vi "Main.vi"() -> ()   [LabVIEW 2017]
uses:
  <userlib>/_NEVSTOP/Communicable State Machine(CSM)/_Polymophic/Add State(s) to Queue By BOOL(Element).vi
  9fd6aee3-8c61-4172-ac23-ecfb0dc55d82.vi
  757b7255-c684-43ce-af59-1acc32dadd6e.vi
  <vilib>/Analysis/2dsp.llb/Real FFT.vi
  <userlib>/_NEVSTOP/Communicable State Machine(CSM)/_Support/CSMQ/_Obtain CSMQ.vi
  <userlib>/_NEVSTOP/Communicable State Machine(CSM)/_Support/FGV-BroadcastRegistry/Cache-Broadcast Registry Search Result.vi
  <userlib>/_NEVSTOP/Communicable State Machine(CSM)/AdvanceAPI/CSM - Unregister Status Change.vi
  <userlib>/_NEVSTOP/Communicable State Machine(CSM)/_Support/CSMQ/_Create Resp Queue.vi
  <userlib>/_NEVSTOP/Communicable State Machine(CSM)/_Support/CSMQ/_Unlock CSMQ.vi
  <userlib>/_NEVSTOP/Communicable State Machine(CSM)/_Support/CSMQ/_Lock State CSMQ.vi
  <userlib>/_NEVSTOP/Communicable State Machine(CSM)/_Support/CSMQ/_Release CSMQ.vi
  <userlib>/_NEVSTOP/Communicable State Machine(CSM)/AdvanceAPI/CSM - Make String Arguments Safe.vi
  <userlib>/_NEVSTOP/Communicable State Machine(CSM)/_Support/CSMQ/_Input Name to CSM Mode.vi
  <userlib>/_NEVSTOP/Communicable State Machine(CSM)/Utility/uuid.vi
  <userlib>/_NEVSTOP/Communicable State Machine(CSM)/_Support/KeyWords.vi
  <userlib>/_NEVSTOP/Communicable State Machine(CSM)/_Support/FGV-BroadcastRegistry/FGV-BroadcastRegistry.vi
  MassData-Parameter/_support/FGV-MassData.vi
  <userlib>/_NEVSTOP/Communicable State Machine(CSM)/_Support/GlobalEvent/FGV-GlobalEventRef.vi
  <userlib>/_NEVSTOP/Communicable State Machine(CSM)/_Support/CSMQ/_CSMQFGV.vi
  <userlib>/_NEVSTOP/Communicable State Machine(CSM)/_Support/CSMQ/_Dequeue CSMQ.vi
  <userlib>/_NEVSTOP/Communicable State Machine(CSM)/_Support/CSMQ/_Enqueue CSMQ.vi
  <userlib>/_NEVSTOP/Communicable State Machine(CSM)/_Support/GlobalEvent/FGV-StatusChangeEventRef.vi
  <userlib>/_NEVSTOP/Communicable State Machine(CSM)/_Support/FGV-BroadcastRegistry/global-Broadcast Cache Change Flag.vi
  MassData-Parameter/JKISM++ MassData Parameter Support.lvlib
  <vilib>/Analysis/NI_AALPro.lvlib
  <userlib>/_NEVSTOP/Communicable State Machine(CSM)/Communicable State Machine.lvlib
panel:
  out "fft":dbl[](graph)
  out "read":cluster{dbl, dbl}(slide)={0.0, 6224.489795918367} scale=0.0..1000000.0 scale format="%#_6p"
  out "Write":cluster{dbl, dbl}(slide)={0.0, 6224.489795918367} scale=0.0..1000000.0 scale format="%#_6p"
  in  "Gen?":bool
  in  "DataSize":i32=1000
  out "Waveform Chart":dbl[](graph)
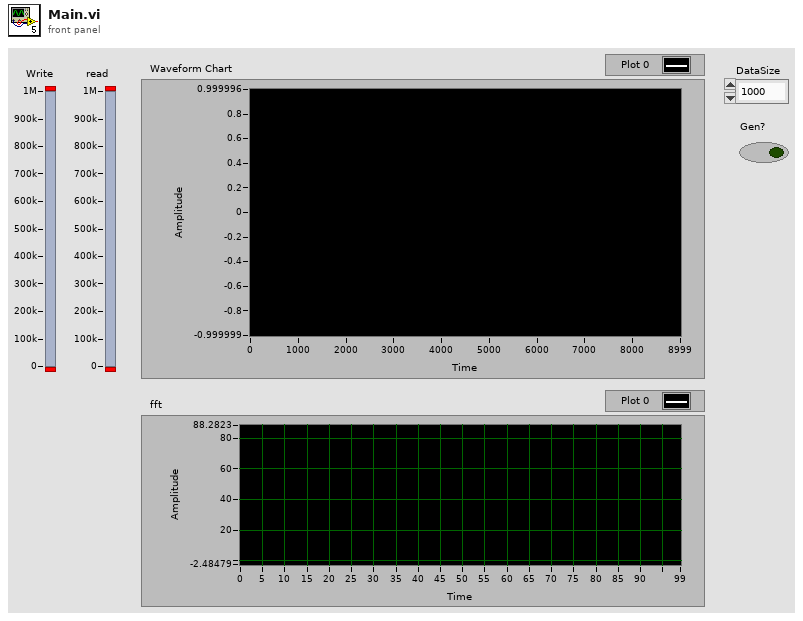
[diagram p1: front panel]
types:
  T1 = enum32{"Invalid", "Standard", "Closed", "Hidden", "Minimized", "Maximized"}
  T2 = enum32{"invalid app kind", "Development System", "Run Time System", "Student Edition", "Embedded LabVIEW", "Evaluation", "Custom"}
  T3 = cluster{"Core":cluster{"Current VI Reference":refnum<vi>, "Close Panel on Exit?":bool}, "Your Boolean data":bool, "Your string data":string}
  T4 = cluster{"Current VI Reference":refnum<vi>, "Close Panel on Exit?":bool}
  T5 = typedef "JKISM++ MassData Parameter Support.lvlib/Def-MassDataOper-Status.ctl" = cluster{"Start":i32, "Size":i32, "Total":i32}
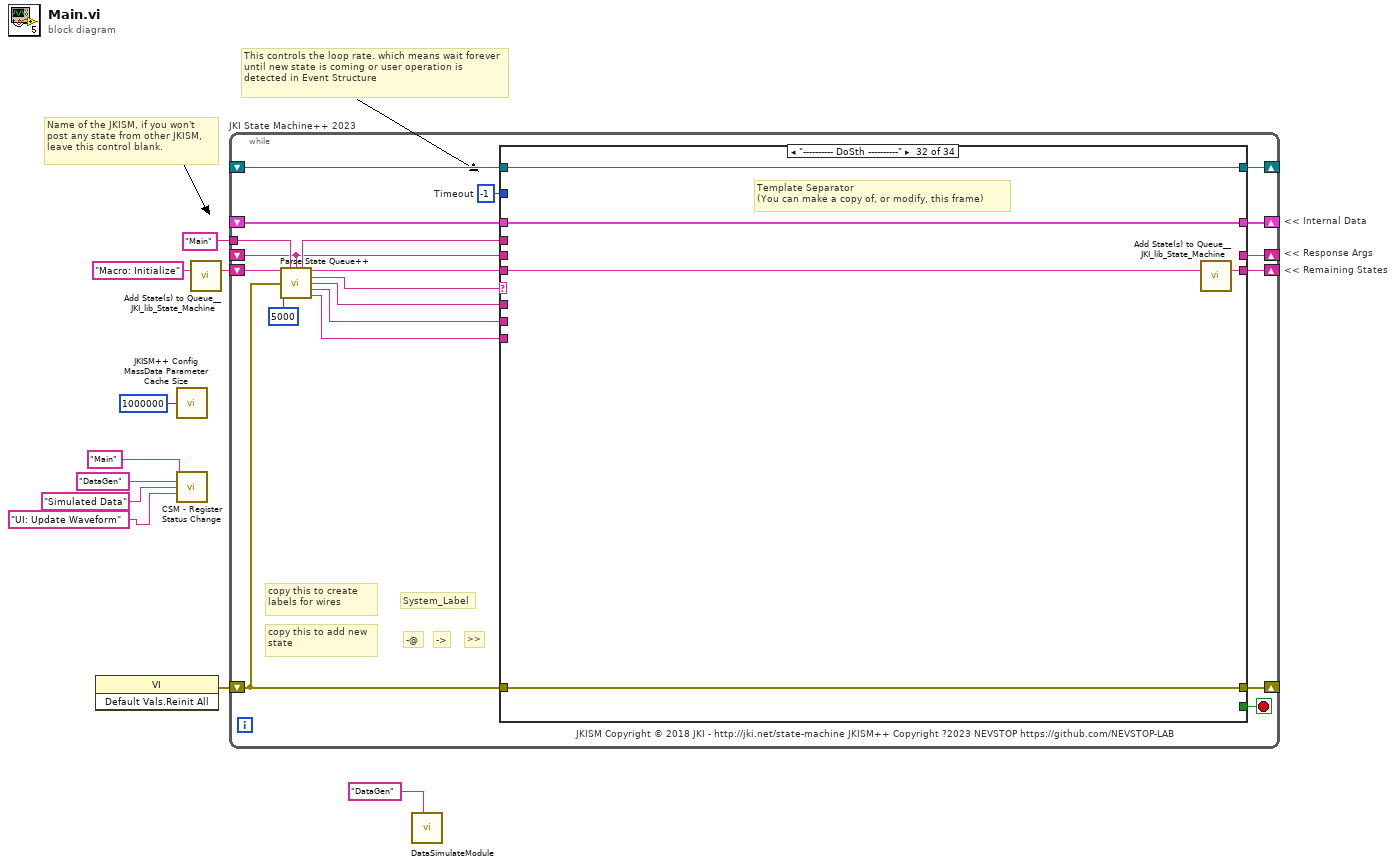
[diagram p0: block diagram]
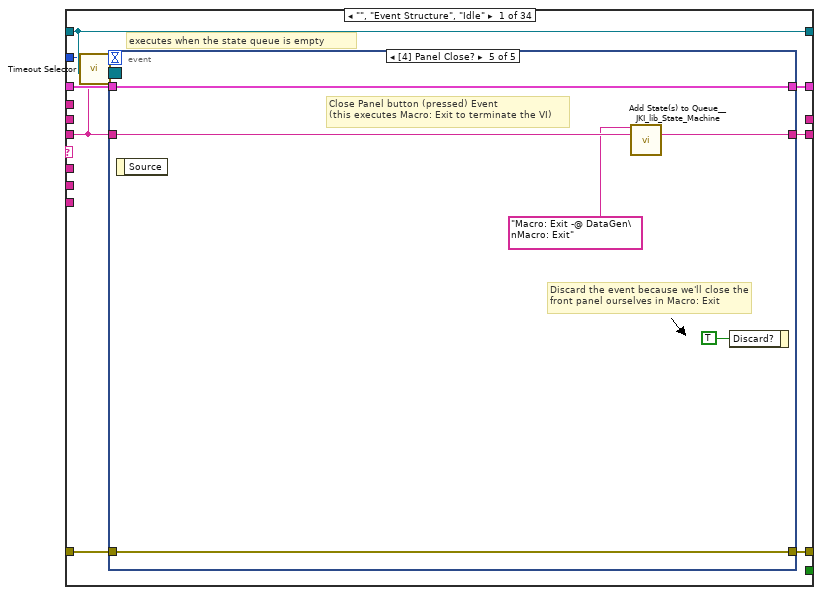
[diagram p2: hidden frame]
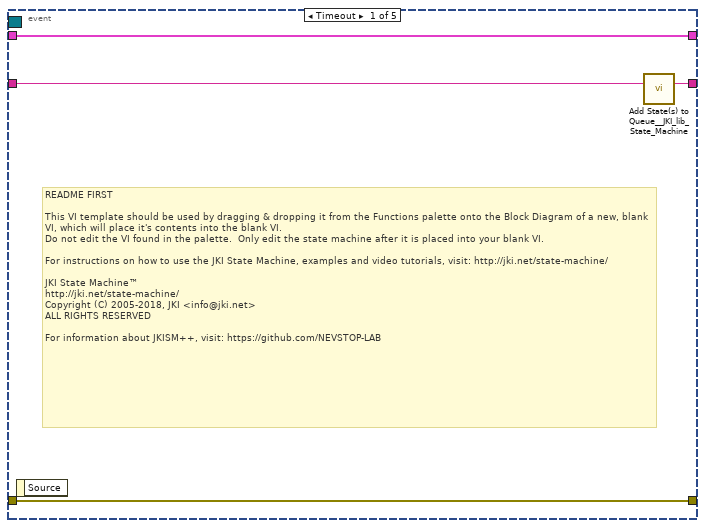
[diagram p3: hidden frame]
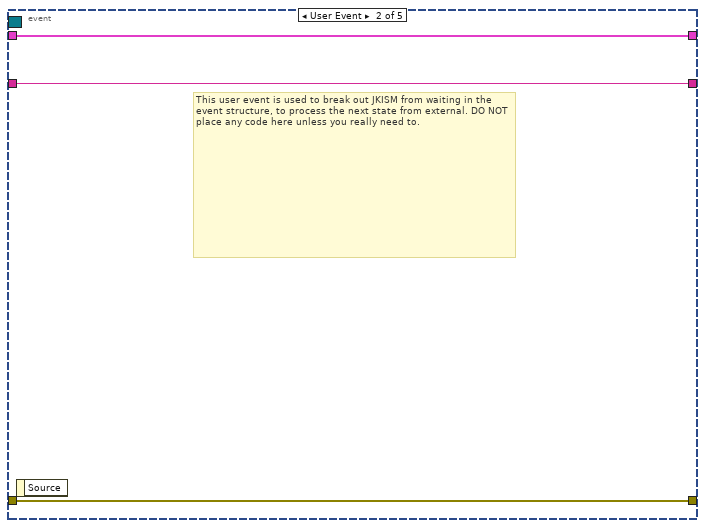
[diagram p4: hidden frame]
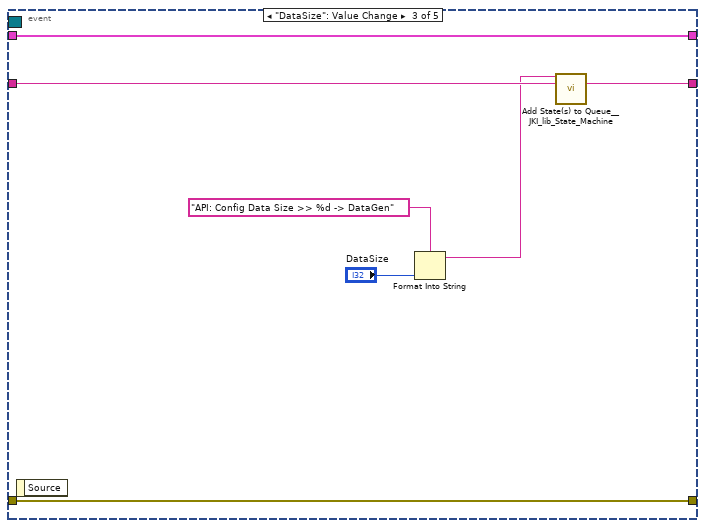
[diagram p5: hidden frame]
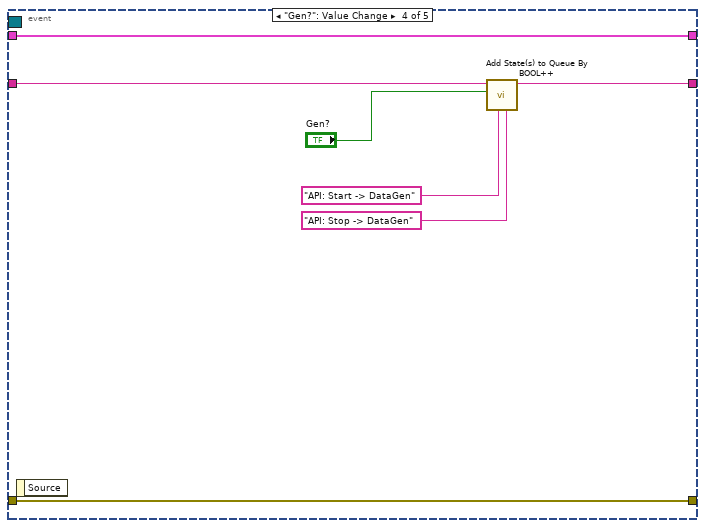
[diagram p6: hidden frame]
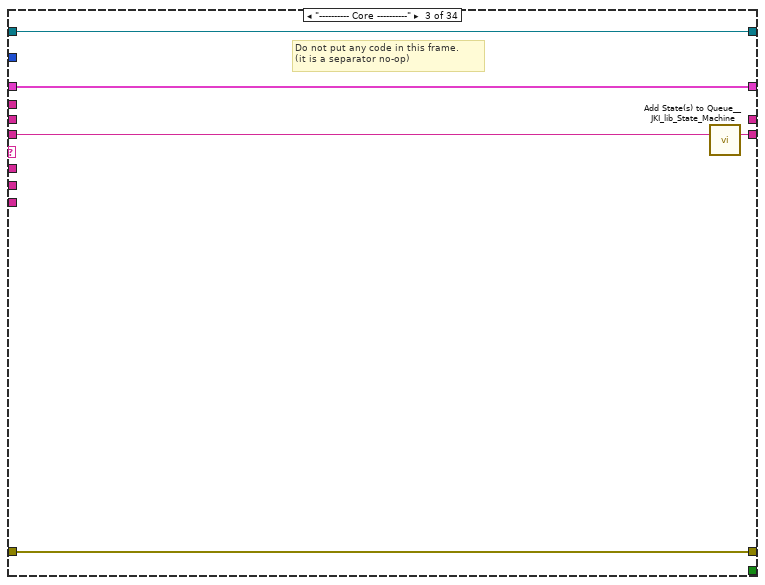
[diagram p8: hidden frame]
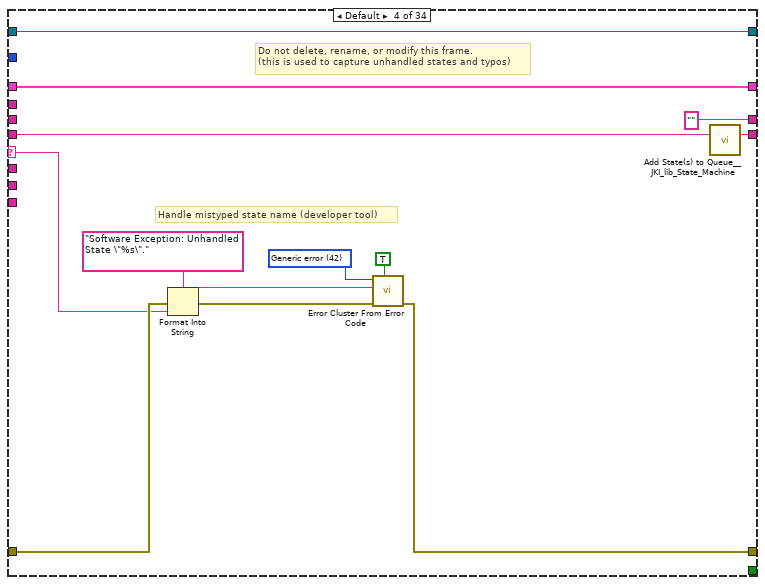
[diagram p9: hidden frame]
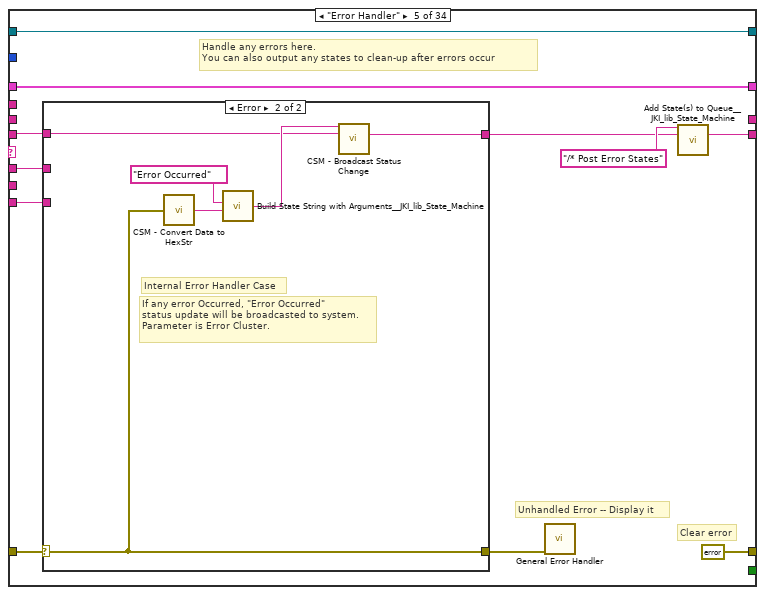
[diagram p10: hidden frame]
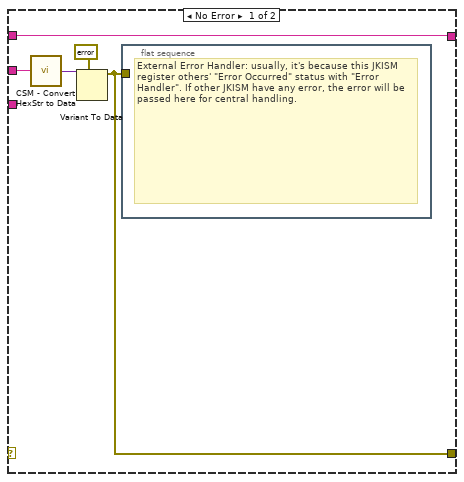
[diagram p11: hidden frame]
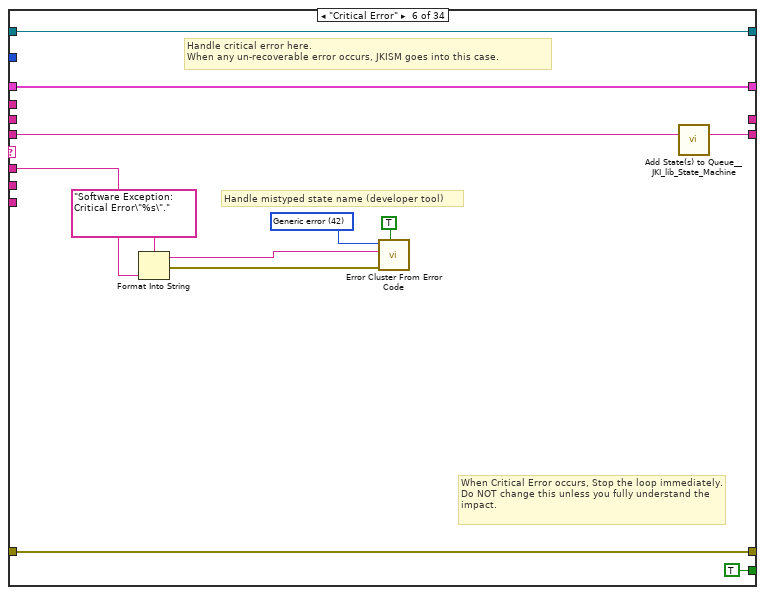
[diagram p12: hidden frame]
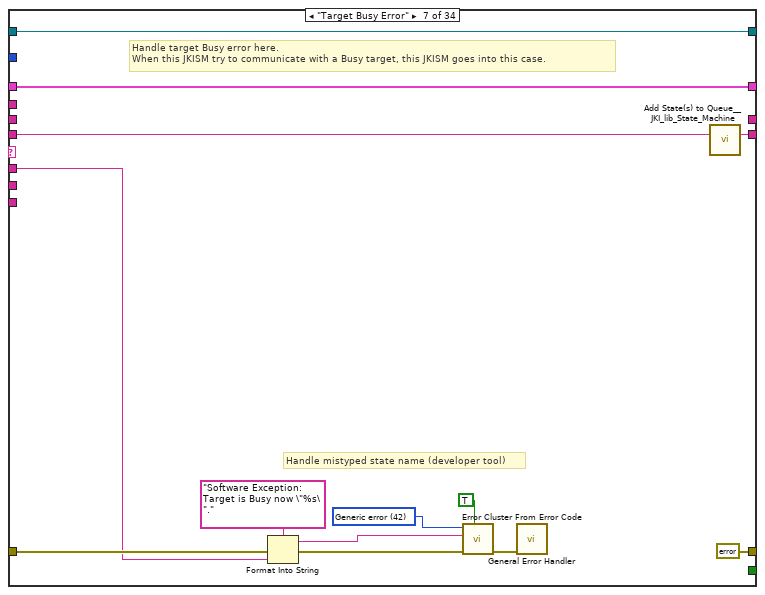
[diagram p13: hidden frame]
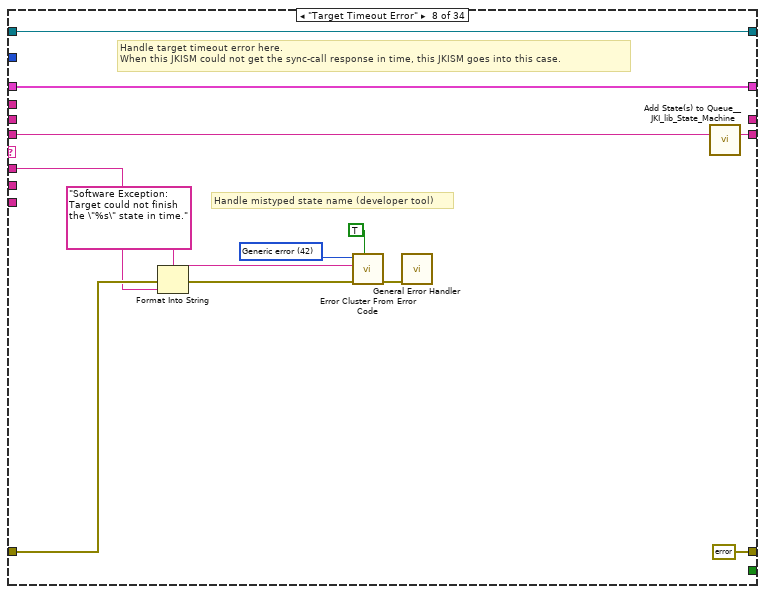
[diagram p14: hidden frame]
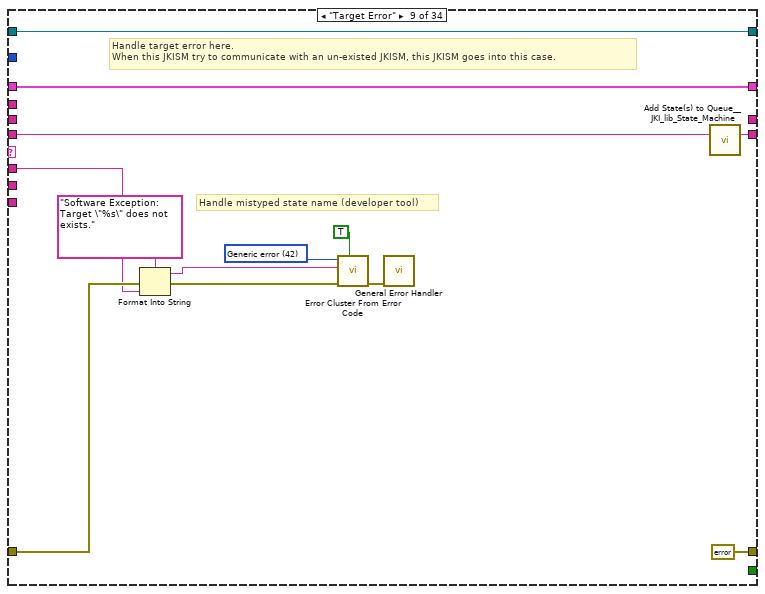
[diagram p15: hidden frame]
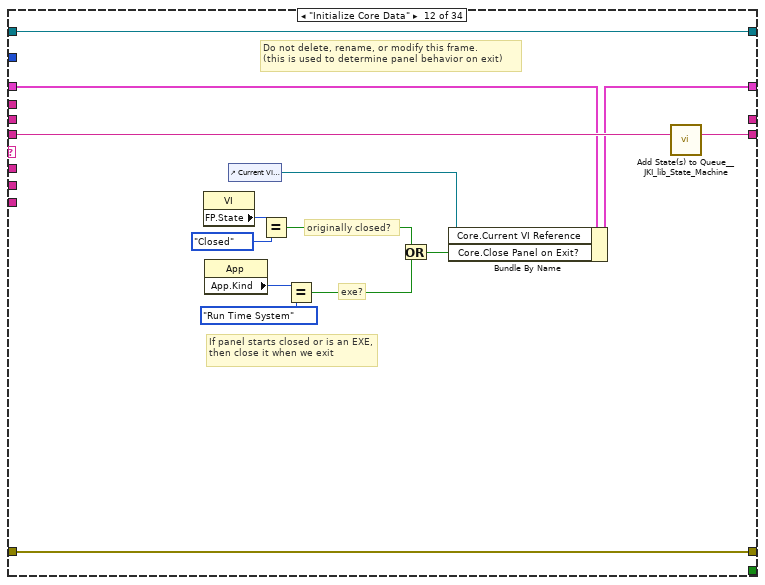
[diagram p18: hidden frame]
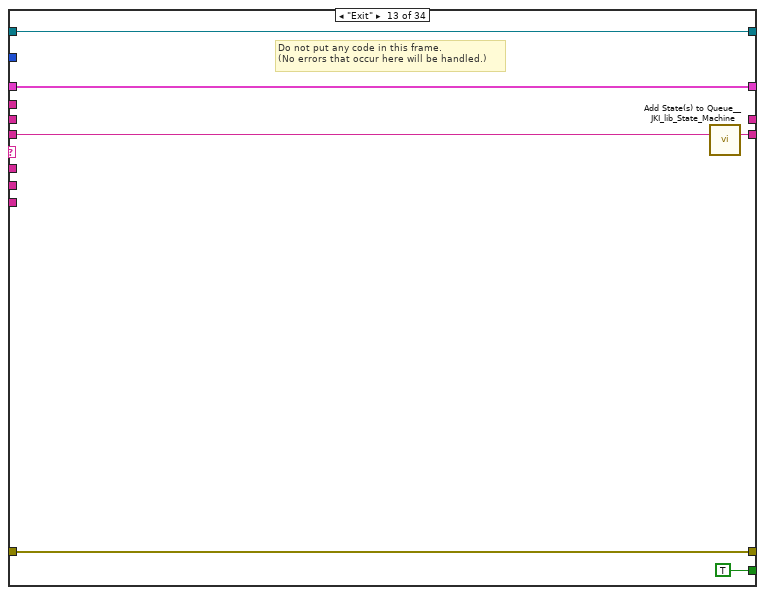
[diagram p19: hidden frame]
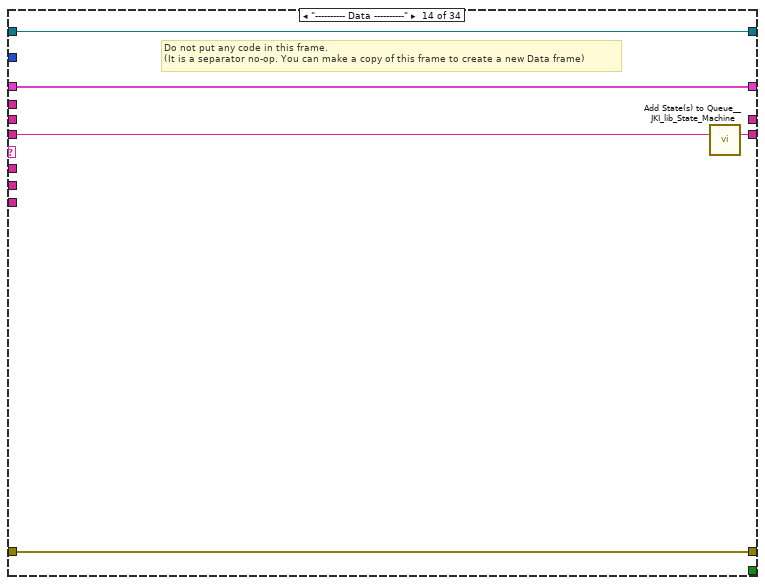
[diagram p20: hidden frame]
diagram:
  # "<< Internal Data"
  # "<< Response Args"
  # "<< Remaining States"
  # "Name of the JKISM, if you won't post any state from other JKISM,  leave this control blank."
  # "This controls the loop rate. which means wait forever until new state is coming or user operation is detected in Event Structure"
  n1 = invoke class="VI" method="Default Vals.Reinit All"() -> (error out=w2:errorcluster)  [unwired: 3 in, 2 out]
  n2 = call "JKISM++ Config MassData Parameter Cache Size.vi"("size(1M)"=1000000) -> ()  [unwired: 9 in]
  n3 = call <userlib>:"CSM - Register Status Change.vi"("CSM Name"="Main" ("JKISM Name"), "Source CSM Name (* as Default)"="DataGen" ("JKISM Name"), "Status"="Simulated Data" ("JKISM Name"), "Response Message (if \"\", same as Source Message)"="UI: Update Waveform" ("JKISM Name")) -> ()  [unwired: 10 in, 2 out]
  n4 = call <vilib>:"Add State(s) to Queue__JKI_lib_State_Machine.vi"("State(s) in (\"\")"="Macro: Initialize") -> ("States Out"=w8:string)  [unwired: 14 in]
  n5 = while "JKI State Machine++ 2023" {
    shift-right: [w25] -> _
    shift-left: _ -> [w24]
    shift-right: [w28] -> _
    shift-left: w2 -> [w22]
    shift-right: [w27] -> _
    shift-left: w8 -> [w29]
    tunnel: "Main" ("Name(\"\" to use uuid)") -> [w17]
    shift-right: [w20] -> _
    shift-left: _ -> [w12]
    shift-right: [w19] -> _
    shift-left: _ -> [w18]
    stop <- w26 stop-if-true
    w23 = -1  # Timeout
    # "JKISM Copyright © 2018 JKI - http://jki.net/state-machine JKISM++ Copyright ?2023 NEVSTOP https://github.com/NEVSTOP-LAB"
    # "copy this to add new state"
    # ">>"
    # "->"
    # "-@"
    # "copy this to create labels for wires"
    # "System_Label"
    n6 = call <userlib>:"Parse State Queue++.vi"("State Queue"=w29, "Name(\"\" to use uuid)"=w17, "Response Arguments"=w12, "Error In (no error)"=w22, "Response Timeout(5000ms)"=5000 ("Response Timeout(1000ms)")) -> ("Name Used"=w13:string, "Remaining States"=w30:string, "Current State"=w16:string, "Arguments"=w11:string, "Argument - State"=w15:string, "From Who"=w14:string)  [unwired: 5 in]
    n7 = case shown="\"---------- DoSth ----------\"" w16 {
      selector: w16 -> [_ _ _ w78 _ _ _ _ _ _ _ _ _ _ _ _ _ _ _ _ _ _ _ _ _ _ _ _ _ _ _ _ _ _]
      tunnel: w30 -> [w31 w69 w75 w82 w92 w120 w125 w143 w156 w164 w168 w183 w189 w194 w202 w209 w214 w220 w224 w230 w240 w247 w263 w334 w352 w361 w367 w373 w384 w387 w392 w398 w404 w410]
      tunnel: w11 -> [_ _ _ _ w90 w113 w127 w139 w152 _ _ _ _ _ _ _ _ _ _ _ _ w242 w257 w329 _ w358 _ _ _ _ _ _ _ _]
      tunnel: w24 -> [w38 w68 w72 w80 w98 w121 w129 w141 w154 w163 w167 w176 w187 w191 _ w204 w211 w219 w223 w227 w238 w245 w259 w338 w351 w360 w364 w370 w381 w386 w391 w395 w401 w407]
      tunnel: [w37 w70 w73 w84 errorcluster {"status"=FALSE, "code"=0, "source"=""} ("error out") w122 errorcluster {"status"=FALSE, "code"=0, "source"=""} ("error out") errorcluster {"status"=FALSE, "code"=0, "source"=""} ("error out") errorcluster {"status"=FALSE, "code"=0, "source"=""} ("error out") w165 w169 w180 w186 w192 w199 w205 w212 w215 w222 w228 w237 w243 w260 w339 w353 w362 w365 w371 w382 w388 w393 w396 w402 w408] -> w28
      tunnel: w22 -> [w36 w70 w73 w83 w96 w122 w131 w144 w157 w165 w169 w180 w186 w192 w199 w206 w212 _ w225 w228 w237 w244 w261 w339 w353 w362 w365 w371 w382 w388 w393 w396 w402 w408]
      tunnel: [w39 w69 w74 w81 w94 w119 w130 w142 w155 w164 w168 w182 w188 w193 w201 w208 w213 w220 w224 w229 w239 w246 w262 w335 w352 w361 w366 w372 w383 w387 w392 w397 w403 w409] -> w27
      tunnel: [_ _ _ _ _ TRUE _ _ _ _ _ _ TRUE _ _ _ _ _ _ _ _ _ _ _ _ _ _ _ _ _ _ _ _ _] -> w26
      tunnel: [w35 w68 w72 w80 w98 w121 w129 w141 w154 w163 w167 w181 w187 w191 w200 w204 w211 w219 w223 w227 w238 w245 w259 w338 w351 w360 w364 w370 w381 w386 w391 w395 w401 w407] -> w25
      tunnel: w23 -> [w33 _ _ _ _ _ _ _ _ _ _ _ _ _ _ _ _ _ _ _ _ _ _ _ _ _ _ _ _ _ _ _ _ _]
      tunnel: w14 -> [_ _ _ _ w89 _ _ _ _ _ _ _ _ _ _ _ _ _ _ _ _ _ _ _ _ _ _ _ _ _ _ _ _ _]
      tunnel: w15 -> [_ _ _ _ _ _ _ _ _ _ _ _ _ _ _ _ _ _ _ _ _ _ _ _ _ _ _ _ _ _ _ _ _ _]
      tunnel: [_ _ _ "" _ _ _ _ _ _ _ _ _ _ _ _ _ _ _ _ _ _ _ _ _ _ _ _ _ _ "API1 Response" _ "DoA Finished" "DoB Finished"] -> w20
      tunnel: [w34 w67 w71 w76 w97 w111 w126 w138 w151 w162 w166 w170 w184 w190 w195 w203 w210 w218 w221 w226 w236 w241 w256 w337 w350 w359 w363 w368 w374 w385 w390 w394 w400 w406] -> w19
      tunnel: w18 -> [w34 w67 w71 w76 w97 w111 w126 w138 w151 w162 w166 w170 w184 w190 w195 w203 w210 _ w221 w226 w236 w241 w256 w337 w350 w359 w363 w368 w374 w385 w390 w394 w400 w406]
      tunnel: w13 -> [_ _ _ _ _ _ _ _ _ _ _ _ _ _ _ _ _ w217 _ _ _ _ _ _ _ _ _ _ _ _ _ _ _ _]
      tunnel: w12 -> [_ _ _ _ _ _ _ _ _ _ _ _ _ _ _ _ _ _ _ _ _ _ _ _ _ _ _ _ _ _ _ _ _ _]
      frame "", "Event Structure", "Idle" {
        # "executes when the state queue is empty"
        n8 = call <userlib>:"Timeout Selector.vi"("Remaining States"=w31, "Timeout Expected"=w33) -> ("Timeout"=w32:i32)  [unwired: 5 in]
        n9 = event shown="[4] Panel Close?" {
          selector: w34 -> [_ _ _ _ _]
          dyn-events: _ -> [_ _ _ _ _]
          timeout: w32 -> [_ _ _ _ _]
          tunnel: w31 -> [w43 w45 w50 w57 w66]
          tunnel: [w42 w45 w51 w58 w65] -> w39
          tunnel: w38 -> [w40 w46 w52 w59 w63]
          tunnel: [w41 w44 w53 w60 w64] -> w37
          tunnel: w36 -> [w41 w44 w53 w60 w64]
          tunnel: [w40 w46 w52 w59 w63] -> w35
          event Timeout {
            # "README FIRST\n \nThis VI template should be used by dragging & dropping it from the Functions palette onto the Block Diagram of a new, blank VI, which will place it's contents into the blank VI. \nDo not edit the VI found in the palette.  Only edit the state machine after it is placed into your blank VI.\n \nFor instructions on how to use the JKI State Machine, examples and video tutorials, visit: http://jki.net/state-machine/\n\nJKI State Machine™\nhttp://jki.net/state-machine/\nCopyright (C) 2005-2018, JKI <info@jki.net>\nALL RIGHTS RESERVED\n\nFor information about JKISM++, visit: https://github.com/NEVSTOP-LAB"
            n10 = event-data() -> ()  [unwired: 1 in, 1 out]
            n11 = call <vilib>:"Add State(s) to Queue__JKI_lib_State_Machine.vi"("State(s) in (\"\")"=w43) -> ("States Out"=w42:string)  [unwired: 14 in]
          }
          event User Event {
            # "This user event is used to break out JKISM from waiting in the event structure, to process the next state from external. DO NOT place any code here unless you really need to."
            n12 = event-data() -> ()  [unwired: 1 in, 1 out]
          }
          event "DataSize": Value Change {
            n13 = event-data() -> ()  [unwired: 1 in, 1 out]
            n14 = Format Into String(format string="API: Config Data Size >> %d -> DataGen" ("State(s) in Front (\"\")"), "DataSize") -> (resulting string=w48:string)  [unwired: 2 in, 1 out]
            n15 = call <vilib>:"Add State(s) to Queue__JKI_lib_State_Machine.vi"("State(s) in Front (\"\")"=w48, "State(s) in (\"\")"=w50) -> ("States Out"=w51:string)  [unwired: 13 in]
          }
          event "Gen?": Value Change {
            n16 = event-data() -> ()  [unwired: 1 in, 1 out]
            n17 = call-poly <userlib>:"Add State(s) to Queue By BOOL++.vi"("False(\"\")"="API: Stop -> DataGen" ("TRUE(\"\")"), "TRUE(\"\")"="API: Start -> DataGen" ("TRUE(\"\")"), "Bool"="Gen?", "State Queue(\"\")"=w57) -> ("State Queue Out"=w58:string)  [unwired: 7 in]
          }
          event Panel Close? {
            # "Discard the event because we'll close the front panel ourselves in Macro: Exit"
            # "Close Panel button (pressed) Event\n(this executes Macro: Exit to terminate the VI)"
            n18 = event-data() -> ()  [unwired: 1 in, 1 out]
            n19 = call <vilib>:"Add State(s) to Queue__JKI_lib_State_Machine.vi"("State(s) in Front (\"\")"="Macro: Exit -@ DataGen\nMacro: Exit", "State(s) in (\"\")"=w66) -> ("States Out"=w65:string)  [unwired: 13 in]
            n20 = event-data("Discard?"=TRUE) -> ()  [unwired: 1 in, 1 out]
          }
        }
      }
      frame "JKISM++ Documentation" {
        # "JKISM++ Documentation"
        # "State Syntax:\nStateCategory: State >> Argument -@ JKISMName\nStateCategory: State >> Argument -> JKISMName\n\nLine Terminator: Line feed"
        # "Commenting:\nTo add a comment use \"//\" or \"#\" and all text to the right will be ignored\nCommenting Example:\nUI: Initialize // This initializes the UI\n// Another comment line"
        # "Example:\nUI: Help >> About -@Main\nUI: Help >> About ->Main\n\nWhere \"UI\" is the state category\nWhere \"Help\" is the state\nWhere \"About\" is the argument\nWhere \"Main\" is the Name of JKISM,which actually run the \"UI: Help >> About\"\n\n    \"-@\" stands for sync state. Current JKISM will wait until the state is finished. \n            - if \"Main\" named JKISM does not exist, \"Target Error\" will occur.\n            - if \"Main\" named JKISM is in another sync remote state, \"Target Busy Error\" will occur.\n            - if \"Main\" named JKISM could not finish the state in time, \"Target Timeout Error\" will occur.\n            - if everything is right. \"Response\" will occur with Argument back from \"Main\" named JKISM. \n\n    \"->\" stands for async state. Current JKISM will post the state and continue to next state in next iteration.\n            - if \"Main\" named JKISM does not exist, \"Target Error\" will occur.\n            - if everything is right. \"Async Message Posted\" will occur.\n            - After State is finished. Caller will receive a \"Async Response\" state from callee.\n\nWhen duplicated name is used for multiple JKISM module or some framework problem happens, \"Critical Error\" will occur."
      }
      frame "---------- Core ----------" {
        # "Do not put any code in this frame.\n(it is a separator no-op)"
        n21 = call <vilib>:"Add State(s) to Queue__JKI_lib_State_Machine.vi"("State(s) in (\"\")"=w75) -> ("States Out"=w74:string)  [unwired: 14 in]
      }
      frame Default {
        w87 = 42 items=["No error", "Argument error", "Memory is full", "Out of zone", "End of file", "File already open", "Generic file I/O error", "File not found", "File permission error", "Disk is full", "Duplicate path", "Too many files open", "System feature not enabled", "Resource file not found", "Cannot add resource", "Resource not found", "Image not found", "Image memory error", "Pen does not exist", "Config type invalid", "Config token not found", "Config parse error", "Config memory error", "Bad external code format", "Bad external code offset", "External code not present", "Null window", "Destroy window error", "Null menu", "Print aborted", "Bad print record", "Print driver error", "Windows error during printing", "Memory error during printing", "Print dialog error", "Generic print error", "Invalid device refnum", "Device not found", "Device parameter error", "Device unit error", "Cannot open device", "Device call aborted", "Generic error", "Cancelled by user", "Object ID too low", "Object ID too high", "Object not in heap", "Unknown heap", "Unknown object (invalid DefProc)", "Unknown object (DefProc not in table)", "Message out of range", "Invalid (null) method", "Unknown message", "Manager call not supported", "Bad address", "Network operation in progress", "Network operation timed out", "Connection is busy", "Network attribute not supported", "Network error", "Address in use", "System out of memory", "Connection aborted", "Connection refused", "Not connected", "Already connected", "Connection closed", "Initialization error (interapplication manager)", "Bad occurrence", "Wait on unbound occurrence handler", "Occurrence queue overflow", "Datalog type conflict", "Unused", "Unrecognized type (interapplication manager)", "Memory corrupt", "Failed to make temporary DLL", "Old CIN version", "Drag socket not found", "Failed to load drop-object", "Failed to register OLE object", "Failed to release OLE object", "Format specifier type mismatch", "Unknown format specifier", "Too few format specifiers", "Too many format specifiers", "Scan failed", "Newer CIN version", "Error converting to variant", "Runtime menu error", "Password tampered", "Variant attribute not found", "Incompatible variant data type", "Event data is not available", "Event Store is not present", "Occurrence is not found", "Event Queue is not created", "Event info is not available", "Refnum passed is NULL", "Error retrieving Class GUID", "Error retrieving CoClass GUID", "Error retrieving TypeLib GUID.", "Bad built application magic bytes.", "Specific driver is different from the specific driver associated with the Logical Name.", "There is no session opened to the class driver.", "Max Error", "MAX - Error with config objects", "MAX - Error loading configuration", "MAX - Group not supported"]
        # "Do not delete, rename, or modify this frame.\n(this is used to capture unhandled states and typos)"
        # "Handle mistyped state name (developer tool)"
        n22 = Format Into String(format string="Software Exception: Unhandled State \"%s\"." ("message"), error in=w83, w78) -> (resulting string=w86:string, error out=w85:errorcluster)  [unwired: 1 in]
        n23 = call <vilib>:"Error Cluster From Error Code.vi"("show call chain? (False)"=TRUE, "error in (no error)"=w85, "error message (\"\")"=w86, "error code (0)"=w87) -> ("error out"=w84:errorcluster)  [unwired: 5 in]
        n24 = call <vilib>:"Add State(s) to Queue__JKI_lib_State_Machine.vi"("State(s) in (\"\")"=w82) -> ("States Out"=w81:string)  [unwired: 14 in]
      }
      frame "Error Handler" {
        # "Unhandled Error -- Display it"
        # "Handle any errors here.\nYou can also output any states to clean-up after errors occur"
        # "Clear error"
        n25 = case shown="Error" w96 {
          selector: w96 -> [_ w105]
          tunnel: [w101 w107] -> w93
          tunnel: w92 -> [w101 w106]
          tunnel: [w100 w105] -> w91
          tunnel: w90 -> [w102 _]
          tunnel: w89 -> [_ _]
          frame No Error {
            n26 = call <userlib>:"CSM - Convert HexStr to Data.vi"("HEX String"=w102) -> ("Variant"=w104:variant)  [unwired: 7 in, 1 out]
            n27 = Variant To Data(type=errorcluster {"status"=FALSE, "code"=0, "source"=""} ("error in (no error)"), Variant=w104) -> (data=w100:errorcluster)  [unwired: 1 in, 1 out]
            n28 = flat-sequence {
              tunnel: w100 -> [_]
              frame #0 {
                # "External Error Handler: usually, it's because this JKISM register others' \"Error Occurred\" status with \"Error Handler\". If other JKISM have any error, the error will be passed here for central handling."
              }
            }
          }
          frame Error {
            # "Internal Error Handler Case"
            # "If any error Occurred, \"Error Occurred\" \nstatus update will be broadcasted to system.\nParameter is Error Cluster."
            n29 = call <userlib>:"CSM - Convert Data to HexStr.vi"("Variant"=w105) -> ("HEX String (0-9,A-F)"=w109:string)  [unwired: 8 in]
            n30 = call <vilib>:"Build State String with Arguments__JKI_lib_State_Machine.vi"("Arguments (\"\")"=w109, "State"="Error Occurred" ("Status with Arguments")) -> ("State with Arguments"=w108:string)  [unwired: 4 in]
            n31 = call <userlib>:"CSM - Broadcast Status Change.vi"("Status with Arguments"=w108, "State Queue"=w106) -> ("Remaining States"=w107:string)  [unwired: 13 in]
          }
        }
        n32 = call <vilib>:"General Error Handler.vi"("error in (no error)"=w91) -> ()  [unwired: 10 in, 5 out]
        n33 = call <vilib>:"Add State(s) to Queue__JKI_lib_State_Machine.vi"("State(s) in Front (\"\")"="/* Post Error States", "State(s) in (\"\")"=w93) -> ("States Out"=w94:string)  [unwired: 13 in]
      }
      frame "Critical Error" {
        w117 = 42 items=["No error", "Argument error", "Memory is full", "Out of zone", "End of file", "File already open", "Generic file I/O error", "File not found", "File permission error", "Disk is full", "Duplicate path", "Too many files open", "System feature not enabled", "Resource file not found", "Cannot add resource", "Resource not found", "Image not found", "Image memory error", "Pen does not exist", "Config type invalid", "Config token not found", "Config parse error", "Config memory error", "Bad external code format", "Bad external code offset", "External code not present", "Null window", "Destroy window error", "Null menu", "Print aborted", "Bad print record", "Print driver error", "Windows error during printing", "Memory error during printing", "Print dialog error", "Generic print error", "Invalid device refnum", "Device not found", "Device parameter error", "Device unit error", "Cannot open device", "Device call aborted", "Generic error", "Cancelled by user", "Object ID too low", "Object ID too high", "Object not in heap", "Unknown heap", "Unknown object (invalid DefProc)", "Unknown object (DefProc not in table)", "Message out of range", "Invalid (null) method", "Unknown message", "Manager call not supported", "Bad address", "Network operation in progress", "Network operation timed out", "Connection is busy", "Network attribute not supported", "Network error", "Address in use", "System out of memory", "Connection aborted", "Connection refused", "Not connected", "Already connected", "Connection closed", "Initialization error (interapplication manager)", "Bad occurrence", "Wait on unbound occurrence handler", "Occurrence queue overflow", "Datalog type conflict", "Unused", "Unrecognized type (interapplication manager)", "Memory corrupt", "Failed to make temporary DLL", "Old CIN version", "Drag socket not found", "Failed to load drop-object", "Failed to register OLE object", "Failed to release OLE object", "Format specifier type mismatch", "Unknown format specifier", "Too few format specifiers", "Too many format specifiers", "Scan failed", "Newer CIN version", "Error converting to variant", "Runtime menu error", "Password tampered", "Variant attribute not found", "Incompatible variant data type", "Event data is not available", "Event Store is not present", "Occurrence is not found", "Event Queue is not created", "Event info is not available", "Refnum passed is NULL", "Error retrieving Class GUID", "Error retrieving CoClass GUID", "Error retrieving TypeLib GUID.", "Bad built application magic bytes.", "Specific driver is different from the specific driver associated with the Logical Name.", "There is no session opened to the class driver.", "Max Error", "MAX - Error with config objects", "MAX - Error loading configuration", "MAX - Group not supported"]
        # "Handle critical error here.\nWhen any un-recoverable error occurs, JKISM goes into this case."
        # "When Critical Error occurs, Stop the loop immediately. Do NOT change this unless you fully understand the impact."
        # "Handle mistyped state name (developer tool)"
        n34 = Format Into String(format string="Software Exception: Critical Error\"%s\"." ("message"), w113) -> (resulting string=w116:string, error out=w115:errorcluster)  [unwired: 2 in]
        n35 = call <vilib>:"Error Cluster From Error Code.vi"("show call chain? (False)"=TRUE, "error in (no error)"=w115, "error message (\"\")"=w116, "error code (0)"=w117) -> ()  [unwired: 5 in, 1 out]
        n36 = call <vilib>:"Add State(s) to Queue__JKI_lib_State_Machine.vi"("State(s) in (\"\")"=w120) -> ("States Out"=w119:string)  [unwired: 14 in]
      }
      frame "Target Busy Error" {
        w134 = 42 items=["No error", "Argument error", "Memory is full", "Out of zone", "End of file", "File already open", "Generic file I/O error", "File not found", "File permission error", "Disk is full", "Duplicate path", "Too many files open", "System feature not enabled", "Resource file not found", "Cannot add resource", "Resource not found", "Image not found", "Image memory error", "Pen does not exist", "Config type invalid", "Config token not found", "Config parse error", "Config memory error", "Bad external code format", "Bad external code offset", "External code not present", "Null window", "Destroy window error", "Null menu", "Print aborted", "Bad print record", "Print driver error", "Windows error during printing", "Memory error during printing", "Print dialog error", "Generic print error", "Invalid device refnum", "Device not found", "Device parameter error", "Device unit error", "Cannot open device", "Device call aborted", "Generic error", "Cancelled by user", "Object ID too low", "Object ID too high", "Object not in heap", "Unknown heap", "Unknown object (invalid DefProc)", "Unknown object (DefProc not in table)", "Message out of range", "Invalid (null) method", "Unknown message", "Manager call not supported", "Bad address", "Network operation in progress", "Network operation timed out", "Connection is busy", "Network attribute not supported", "Network error", "Address in use", "System out of memory", "Connection aborted", "Connection refused", "Not connected", "Already connected", "Connection closed", "Initialization error (interapplication manager)", "Bad occurrence", "Wait on unbound occurrence handler", "Occurrence queue overflow", "Datalog type conflict", "Unused", "Unrecognized type (interapplication manager)", "Memory corrupt", "Failed to make temporary DLL", "Old CIN version", "Drag socket not found", "Failed to load drop-object", "Failed to register OLE object", "Failed to release OLE object", "Format specifier type mismatch", "Unknown format specifier", "Too few format specifiers", "Too many format specifiers", "Scan failed", "Newer CIN version", "Error converting to variant", "Runtime menu error", "Password tampered", "Variant attribute not found", "Incompatible variant data type", "Event data is not available", "Event Store is not present", "Occurrence is not found", "Event Queue is not created", "Event info is not available", "Refnum passed is NULL", "Error retrieving Class GUID", "Error retrieving CoClass GUID", "Error retrieving TypeLib GUID.", "Bad built application magic bytes.", "Specific driver is different from the specific driver associated with the Logical Name.", "There is no session opened to the class driver.", "Max Error", "MAX - Error with config objects", "MAX - Error loading configuration", "MAX - Group not supported"]
        # "Handle target Busy error here.\nWhen this JKISM try to communicate with a Busy target, this JKISM goes into this case."
        # "Handle mistyped state name (developer tool)"
        n37 = Format Into String(format string="Software Exception: Target is Busy now \"%s\"." ("message"), error in=w131, w127) -> (resulting string=w133:string, error out=w132:errorcluster)  [unwired: 1 in]
        n38 = call <vilib>:"Error Cluster From Error Code.vi"("show call chain? (False)"=TRUE, "error in (no error)"=w132, "error message (\"\")"=w133, "error code (0)"=w134) -> ("error out"=w124:errorcluster)  [unwired: 5 in]
        n39 = call <vilib>:"General Error Handler.vi"("error in (no error)"=w124) -> ()  [unwired: 10 in, 5 out]
        n40 = call <vilib>:"Add State(s) to Queue__JKI_lib_State_Machine.vi"("State(s) in (\"\")"=w125) -> ("States Out"=w130:string)  [unwired: 14 in]
      }
      frame "Target Timeout Error" {
        w147 = 42 items=["No error", "Argument error", "Memory is full", "Out of zone", "End of file", "File already open", "Generic file I/O error", "File not found", "File permission error", "Disk is full", "Duplicate path", "Too many files open", "System feature not enabled", "Resource file not found", "Cannot add resource", "Resource not found", "Image not found", "Image memory error", "Pen does not exist", "Config type invalid", "Config token not found", "Config parse error", "Config memory error", "Bad external code format", "Bad external code offset", "External code not present", "Null window", "Destroy window error", "Null menu", "Print aborted", "Bad print record", "Print driver error", "Windows error during printing", "Memory error during printing", "Print dialog error", "Generic print error", "Invalid device refnum", "Device not found", "Device parameter error", "Device unit error", "Cannot open device", "Device call aborted", "Generic error", "Cancelled by user", "Object ID too low", "Object ID too high", "Object not in heap", "Unknown heap", "Unknown object (invalid DefProc)", "Unknown object (DefProc not in table)", "Message out of range", "Invalid (null) method", "Unknown message", "Manager call not supported", "Bad address", "Network operation in progress", "Network operation timed out", "Connection is busy", "Network attribute not supported", "Network error", "Address in use", "System out of memory", "Connection aborted", "Connection refused", "Not connected", "Already connected", "Connection closed", "Initialization error (interapplication manager)", "Bad occurrence", "Wait on unbound occurrence handler", "Occurrence queue overflow", "Datalog type conflict", "Unused", "Unrecognized type (interapplication manager)", "Memory corrupt", "Failed to make temporary DLL", "Old CIN version", "Drag socket not found", "Failed to load drop-object", "Failed to register OLE object", "Failed to release OLE object", "Format specifier type mismatch", "Unknown format specifier", "Too few format specifiers", "Too many format specifiers", "Scan failed", "Newer CIN version", "Error converting to variant", "Runtime menu error", "Password tampered", "Variant attribute not found", "Incompatible variant data type", "Event data is not available", "Event Store is not present", "Occurrence is not found", "Event Queue is not created", "Event info is not available", "Refnum passed is NULL", "Error retrieving Class GUID", "Error retrieving CoClass GUID", "Error retrieving TypeLib GUID.", "Bad built application magic bytes.", "Specific driver is different from the specific driver associated with the Logical Name.", "There is no session opened to the class driver.", "Max Error", "MAX - Error with config objects", "MAX - Error loading configuration", "MAX - Group not supported"]
        # "Handle target timeout error here.\nWhen this JKISM could not get the sync-call response in time, this JKISM goes into this case."
        # "Handle mistyped state name (developer tool)"
        n41 = Format Into String(format string="Software Exception: Target could not finish the \"%s\" state in time." ("message"), error in=w144, w139) -> (resulting string=w146:string, error out=w145:errorcluster)  [unwired: 1 in]
        n42 = call <vilib>:"Error Cluster From Error Code.vi"("show call chain? (False)"=TRUE, "error in (no error)"=w145, "error message (\"\")"=w146, "error code (0)"=w147) -> ("error out"=w136:errorcluster)  [unwired: 5 in]
        n43 = call <vilib>:"General Error Handler.vi"("error in (no error)"=w136) -> ()  [unwired: 10 in, 5 out]
        n44 = call <vilib>:"Add State(s) to Queue__JKI_lib_State_Machine.vi"("State(s) in (\"\")"=w143) -> ("States Out"=w142:string)  [unwired: 14 in]
      }
      frame "Target Error" {
        w160 = 42 items=["No error", "Argument error", "Memory is full", "Out of zone", "End of file", "File already open", "Generic file I/O error", "File not found", "File permission error", "Disk is full", "Duplicate path", "Too many files open", "System feature not enabled", "Resource file not found", "Cannot add resource", "Resource not found", "Image not found", "Image memory error", "Pen does not exist", "Config type invalid", "Config token not found", "Config parse error", "Config memory error", "Bad external code format", "Bad external code offset", "External code not present", "Null window", "Destroy window error", "Null menu", "Print aborted", "Bad print record", "Print driver error", "Windows error during printing", "Memory error during printing", "Print dialog error", "Generic print error", "Invalid device refnum", "Device not found", "Device parameter error", "Device unit error", "Cannot open device", "Device call aborted", "Generic error", "Cancelled by user", "Object ID too low", "Object ID too high", "Object not in heap", "Unknown heap", "Unknown object (invalid DefProc)", "Unknown object (DefProc not in table)", "Message out of range", "Invalid (null) method", "Unknown message", "Manager call not supported", "Bad address", "Network operation in progress", "Network operation timed out", "Connection is busy", "Network attribute not supported", "Network error", "Address in use", "System out of memory", "Connection aborted", "Connection refused", "Not connected", "Already connected", "Connection closed", "Initialization error (interapplication manager)", "Bad occurrence", "Wait on unbound occurrence handler", "Occurrence queue overflow", "Datalog type conflict", "Unused", "Unrecognized type (interapplication manager)", "Memory corrupt", "Failed to make temporary DLL", "Old CIN version", "Drag socket not found", "Failed to load drop-object", "Failed to register OLE object", "Failed to release OLE object", "Format specifier type mismatch", "Unknown format specifier", "Too few format specifiers", "Too many format specifiers", "Scan failed", "Newer CIN version", "Error converting to variant", "Runtime menu error", "Password tampered", "Variant attribute not found", "Incompatible variant data type", "Event data is not available", "Event Store is not present", "Occurrence is not found", "Event Queue is not created", "Event info is not available", "Refnum passed is NULL", "Error retrieving Class GUID", "Error retrieving CoClass GUID", "Error retrieving TypeLib GUID.", "Bad built application magic bytes.", "Specific driver is different from the specific driver associated with the Logical Name.", "There is no session opened to the class driver.", "Max Error", "MAX - Error with config objects", "MAX - Error loading configuration", "MAX - Group not supported"]
        # "Handle target error here.\nWhen this JKISM try to communicate with an un-existed JKISM, this JKISM goes into this case."
        # "Handle mistyped state name (developer tool)"
        n45 = Format Into String(format string="Software Exception: Target \"%s\" does not exists." ("message"), error in=w157, w152) -> (resulting string=w159:string, error out=w158:errorcluster)  [unwired: 1 in]
        n46 = call <vilib>:"Error Cluster From Error Code.vi"("show call chain? (False)"=TRUE, "error in (no error)"=w158, "error message (\"\")"=w159, "error code (0)"=w160) -> ("error out"=w150:errorcluster)  [unwired: 5 in]
        n47 = call <vilib>:"General Error Handler.vi"("error in (no error)"=w150) -> ()  [unwired: 10 in, 5 out]
        n48 = call <vilib>:"Add State(s) to Queue__JKI_lib_State_Machine.vi"("State(s) in (\"\")"=w156) -> ("States Out"=w155:string)  [unwired: 14 in]
      }
      frame "Async Response", "Response" {
        # "Handle Async-call Response (\"Async Response\" for ->)"
        # "Handle Sync-call Response (\"Response\" for -@)"
        # "After Message is executed, JKISM+ goes to this state for receive the response. \n    For Async Message(->), \"Async Response\" is used. This JKISM will goes to \"Async Message Posted\" immediately and receive the \"Async Response\" after the callee finishes the message.\n    For Sync Message(@),  This JKISM will wait until the message is done and immediately goes to \"Response\""
      }
      frame "Async Message Posted" {
        # "Handle post action for async message (->)."
        # "After Async Message is posted (->), JKISM+ goes to this state for post-action. You can use Argument - State to tell which Async Message is called."
      }
      frame "Initialize Core Data" {
        # "Do not delete, rename, or modify this frame.\n(this is used to determine panel behavior on exit)"
        # "originally closed?"
        # "exe?"
        # "If panel starts closed or is an EXE, then close it when we exit"
        n49 = property class="VI"() -> ("FP.State"=w173:T1)  [unwired: 2 in, 2 out]
        n50 = property class="App"() -> ("App.Kind"=w179:T2)  [unwired: 2 in, 2 out]
        n51 = control-ref of="Current VI Reference"() -> (w174:refnum<vi>)
        n52 = Equal?(x=w173, y=T1."Closed" ("Front Panel Window:State")) -> (x = y?=w171:bool)
        n53 = Equal?(x=w179, y=T2."Run Time System" ("Application:Kind")) -> (x = y?=w177:bool)
        n54 = Or(x=w171, y=w177) -> (x .or. y?=w175:bool)
        n55 = Bundle By Name(cluster=w176, "Core.Current VI Reference"=w174, "Core.Close Panel on Exit?"=w175) -> (w181:T3)
        n56 = call <vilib>:"Add State(s) to Queue__JKI_lib_State_Machine.vi"("State(s) in (\"\")"=w183) -> ("States Out"=w182:string)  [unwired: 14 in]
      }
      frame "Exit" {
        # "Do not put any code in this frame.\n(No errors that occur here will be handled.)"
        n57 = call <vilib>:"Add State(s) to Queue__JKI_lib_State_Machine.vi"("State(s) in (\"\")"=w189) -> ("States Out"=w188:string)  [unwired: 14 in]
      }
      frame "---------- Data ----------" {
        # "Do not put any code in this frame.\n(It is a separator no-op. You can make a copy of this frame to create a new Data frame)"
        n58 = call <vilib>:"Add State(s) to Queue__JKI_lib_State_Machine.vi"("State(s) in (\"\")"=w194) -> ("States Out"=w193:string)  [unwired: 14 in]
      }
      frame "Data: Initialize" {
        w196 = T4 {"Current VI Reference"=refnum, "Close Panel on Exit?"=FALSE}  # Core
        w198 = TRUE  # Your Boolean data
        w197 = ""  # Your string data
        # "do not delete - used by framework"
        # "Expand Bundle to add new data elements to shift register data."
        # "Add new data here."
        # "Data names and types of shift register data are defined by this bundle."
        # "Initialize the shift-register data, here.\n(data names are defined by what you wire into the bundle function)"
        n59 = Bundle("Core"=w196, "Your Boolean data"=w198, "Your string data"=w197) -> (w200:T3)  [unwired: 1 in]
        n60 = call <vilib>:"Add State(s) to Queue__JKI_lib_State_Machine.vi"("State(s) in (\"\")"=w202) -> ("States Out"=w201:string)  [unwired: 14 in]
      }
      frame "Data: Cleanup" {
        # "Cleanup any data and references, here.\n(this is called automatically, by the Macro: Exit)"
        n61 = Unbundle By Name(w204) -> ("Core.Current VI Reference"=w207:refnum<vi>)
        n62 = Close Reference(reference=w207, error in (no error)=w206) -> (error out=w205:errorcluster)
        n63 = call <vilib>:"Add State(s) to Queue__JKI_lib_State_Machine.vi"("State(s) in (\"\")"=w209) -> ("States Out"=w208:string)  [unwired: 14 in]
      }
      frame "---------- Events ----------" {
        # "Do not put any code in this frame.\n(It is a separator no-op. You can make a copy of this frame to create a new UI frame)"
        n64 = call <vilib>:"Add State(s) to Queue__JKI_lib_State_Machine.vi"("State(s) in (\"\")"=w214) -> ("States Out"=w213:string)  [unwired: 14 in]
      }
      frame "Events: Register" {
        # "Register message event to break Waiting in Event structure."
        n65 = call <userlib>:"CSM - Get New State Notifier Event.vi"("Name(\"\" to use uuid) in"=w217) -> ("Error out"=w215:errorcluster, "New State Notifier Event"=w216:refnum<user-event>)  [unwired: 9 in]
        n66 = register-events(w216) -> (reference out=w218:refnum<event-registration>)  [unwired: 2 in, 1 out]
      }
      frame "Events: Unregister" {
        n67 = Unregister For Events(event registration refnum=w221, error in=w225) -> (error out=w222:errorcluster)
      }
      frame "---------- UI ----------" {
        # "Do not put any code in this frame.\n(It is a separator no-op. You can make a copy of this frame to create a new UI frame)"
        n68 = call <vilib>:"Add State(s) to Queue__JKI_lib_State_Machine.vi"("State(s) in (\"\")"=w230) -> ("States Out"=w229:string)  [unwired: 14 in]
      }
      frame "UI: Initialize" {
        # "Initialize the User Interface, here.\n(this is called automatically, by the Macro: Init)"
        n69 = call "JKISM++ MassData Parameter Status.vi"() -> ("cache size"=w231:i32)  [unwired: 9 in, 2 out]
        n70 = property on="Write" class="Slide (strict)"("Scale.Maximum"=w231, "Scale.Minimum"=0.0 ("Scale.Range:Minimum"), "Scale.Increment"=1.0 ("Scale.Range:Minor Increment")) -> ()  [unwired: 2 in, 2 out]
        n71 = property on="read" class="Slide (strict)"("Scale.Maximum"=w231, "Scale.Minimum"=0.0 ("Scale.Range:Minimum"), "Scale.Increment"=1.0 ("Scale.Range:Minor Increment")) -> ()  [unwired: 2 in, 2 out]
        n72 = call <vilib>:"Add State(s) to Queue__JKI_lib_State_Machine.vi"("State(s) in (\"\")"=w240) -> ("States Out"=w239:string)  [unwired: 14 in]
      }
      frame "UI: Cursor Set" {
        # "Argument"
        # "Set and Unset Cursor Busy.\n(Usage: \"UI: Cursor Set >> Busy|Idle\")"
        n73 = disable-structure shown="Default" {
          disable-tunnel: w244 -> [w250 w255]
          disable-tunnel: [w249 w255] -> w243
          disable-tunnel: w242 -> [w248 _]
          frame condition #0 (active) {
            n74 = case shown="\"Busy\"" w248 {
              tunnel: w250 -> [w252 w254]
              tunnel: [w251 w253] -> w249
              frame "Idle", Default {
                n75 = call <vilib>:"Unset Busy.vi"("error in (no error)"=w252) -> ("error out"=w251:errorcluster)  [unwired: 10 in]
              }
              frame "Busy" {
                n76 = call <vilib>:"Set Busy.vi"("error in (no error)"=w254) -> ("error out"=w253:errorcluster)  [unwired: 9 in, 1 out]
              }
            }
          }
          frame condition #1 {
          }
        }
        n77 = call <vilib>:"Add State(s) to Queue__JKI_lib_State_Machine.vi"("State(s) in (\"\")"=w247) -> ("States Out"=w246:string)  [unwired: 14 in]
      }
      frame "UI: Front Panel State" {
        # "Argument"
        # "Set Front Panel Open or Closed\n(Usage: \"UI: Front Panel State >> Open|Close\")"
        n78 = Unbundle By Name(w259) -> ("Core.Current VI Reference"=w258:refnum<vi>)
        n79 = case shown="\"Minimize\", \"Minimized\"" w257 {
          tunnel: w261 -> [w269 w284 w295 w308 w321]
          tunnel: [w271 w285 w297 w310 w323] -> w260
          tunnel: w258 -> [w270 w282 w296 w309 w322]
          frame "Open", "Standard", Default {
            w264 = T1."Standard" ("State")
            n80 = property class="VI"(reference=w270, error in=w269) -> (reference out=w267:refnum<vi>, error out=w268:errorcluster, "FP.State"=w266:T1)
            n81 = Not Equal?(x=w266, y=w264) -> (x != y?=w265:bool)
            n82 = case shown="True" w265 {
              tunnel: [w275 w277] -> w271
              tunnel: w268 -> [w274 w277]
              tunnel: w267 -> [w273 _]
              tunnel: w264 -> [w272 _]
              frame True {
                n83 = invoke class="VI" method="FP.Open"(reference=w273, error in=w274, "Activate"=TRUE, "State"=w272) -> (error out=w275:errorcluster)  [unwired: 1 in, 4 out]
              }
              frame False {
              }
            }
          }
          frame "Close", "Closed" {
            n84 = property class="VI"(reference=w282, error in=w284) -> (reference out=w281:refnum<vi>, error out=w283:errorcluster, "FP.State"=w279:T1)
            n85 = Not Equal?(x=w279, y=T1."Closed" ("Front Panel Window:State")) -> (x != y?=w278:bool)
            n86 = case shown="True" w278 {
              tunnel: [w286 w289] -> w285
              tunnel: w283 -> [w286 w288]
              tunnel: w281 -> [_ w287]
              frame False {
              }
              frame True {
                n87 = invoke class="VI" method="FP.Close"(reference=w287, error in=w288) -> (error out=w289:errorcluster)  [unwired: 1 in, 2 out]
              }
            }
          }
          frame "Hidden", "Hide" {
            w290 = T1."Hidden" ("State")
            n88 = property class="VI"(reference=w296, error in=w295) -> (reference out=w293:refnum<vi>, error out=w294:errorcluster, "FP.State"=w292:T1)
            n89 = Not Equal?(x=w292, y=w290) -> (x != y?=w291:bool)
            n90 = case shown="True" w291 {
              tunnel: [w301 w302] -> w297
              tunnel: w294 -> [w300 w302]
              tunnel: w293 -> [w299 _]
              tunnel: w290 -> [w298 _]
              frame True {
                n91 = invoke class="VI" method="FP.Open"(reference=w299, error in=w300, "State"=w298) -> (error out=w301:errorcluster)  [unwired: 2 in, 4 out]
              }
              frame False {
              }
            }
          }
          frame "Minimize", "Minimized" {
            w303 = T1."Minimized" ("State")
            n92 = property class="VI"(reference=w309, error in=w308) -> (reference out=w306:refnum<vi>, error out=w307:errorcluster, "FP.State"=w305:T1)
            n93 = Not Equal?(x=w305, y=w303) -> (x != y?=w304:bool)
            n94 = case shown="True" w304 {
              tunnel: [w314 w315] -> w310
              tunnel: w307 -> [w313 w315]
              tunnel: w306 -> [w312 _]
              tunnel: w303 -> [w311 _]
              frame True {
                n95 = invoke class="VI" method="FP.Open"(reference=w312, error in=w313, "State"=w311) -> (error out=w314:errorcluster)  [unwired: 2 in, 4 out]
              }
              frame False {
              }
            }
          }
          frame "Maximize", "Maximized" {
            w316 = T1."Maximized" ("State")
            n96 = property class="VI"(reference=w322, error in=w321) -> (reference out=w319:refnum<vi>, error out=w320:errorcluster, "FP.State"=w318:T1)
            n97 = Not Equal?(x=w318, y=w316) -> (x != y?=w317:bool)
            n98 = case shown="True" w317 {
              tunnel: [w327 w328] -> w323
              tunnel: w320 -> [w326 w328]
              tunnel: w319 -> [w325 _]
              tunnel: w316 -> [w324 _]
              frame True {
                n99 = invoke class="VI" method="FP.Open"(reference=w325, error in=w326, "State"=w324) -> (error out=w327:errorcluster)  [unwired: 2 in, 4 out]
              }
              frame False {
              }
            }
          }
        }
        n100 = call <vilib>:"Add State(s) to Queue__JKI_lib_State_Machine.vi"("State(s) in (\"\")"=w263) -> ("States Out"=w262:string)  [unwired: 14 in]
      }
      frame "UI: Update Waveform" {
        n101 = call "JKISM++ Convert Argument to MassData.vim"("Type"=dbl[] [], "HEX Argument"=w329) -> ("DBL"=→"Waveform Chart":dbl[])  [unwired: 7 in]
        n102 = call <vilib>:"Build State String with Arguments__JKI_lib_State_Machine.vi"("Arguments (\"\")"=w329, "State"="UI: FFT" ("State(s) in Front (\"\")")) -> ("State with Arguments"=w332:string)  [unwired: 4 in]
        n103 = call <vilib>:"Add State(s) to Queue__JKI_lib_State_Machine.vi"("State(s) in Front (\"\")"=w332, "State(s) in (\"\")"=w334, "State(s) at Back (\"\")"="UI: Update Cache Status" ("State(s) at Back (\"\")")) -> ("States Out"=w335:string)  [unwired: 12 in]
      }
      frame "UI: Update Cache Status" {
        n104 = call "JKISM++ MassData Parameter Status.vi"() -> ("Active Read Oper"=w341:T5, "Active Write Oper"=w345:T5)  [unwired: 9 in, 1 out]
        n105 = Unbundle(w345) -> ("Start"=w348:i32, "Size"=w346:i32)  [unwired: 1 out]
        n106 = Unbundle(w341) -> ("Start"=w342:i32, "Size"=w344:i32)  [unwired: 1 out]
        n107 = Add(x=w348, y=w346) -> (x+y=w347:i32)
        n108 = Add(x=w342, y=w344) -> (x+y=w343:i32)
        n109 = Bundle(w347, "Start"=w348) -> (→"Write":cluster{i32, "Start":i32})  [unwired: 1 in]
        n110 = Bundle(w343, "Start"=w342) -> (→"read":cluster{i32, "Start":i32})  [unwired: 1 in]
      }
      frame "UI: FFT" {
        n111 = call "JKISM++ Convert Argument to MassData.vim"("Type"=dbl[] [], "HEX Argument"=w358) -> ("DBL"=w357:dbl[])  [unwired: 7 in]
        n112 = local read "DataSize"() -> (w356:i32)
        n113 = call-poly <vilib>:"FFT.vi"("FFT size"=w356, "X"=w357) -> ("FFT {X}"=→"fft":cdb[])  [unwired: 8 in, 1 out]
      }
      frame "---------- Macro ----------" {
        # "Do not put any code in this frame.\n(It is a separator no-op. You can make a copy of this frame to create a new Macro frame)"
        n114 = call <vilib>:"Add State(s) to Queue__JKI_lib_State_Machine.vi"("State(s) in (\"\")"=w367) -> ("States Out"=w366:string)  [unwired: 14 in]
      }
      frame "Macro: Initialize" {
        w369 = "Data: Initialize\nInitialize Core Data\nEvents: Register\nUI: Initialize\nUI: Front Panel State >> Open"  # Data: Initialize Initialize Core Data Events: Register UI: Initialize UI: Front Panel State >> Open
        # "Initialization Macro\n(This is called once, when the VI starts)"
        n115 = call <vilib>:"Add State(s) to Queue__JKI_lib_State_Machine.vi"("State(s) in Front (\"\")"=w369, "State(s) in (\"\")"=w373) -> ("States Out"=w372:string)  [unwired: 13 in]
      }
      frame "Macro: Exit" {
        # "Exit Macro\n(This is called once, when the VI exits)"
        n116 = Unbundle By Name(w381) -> ("Core.Close Panel on Exit?"=w380:bool)
        n117 = Select(t="UI: Front Panel State >> Close", s=w380, f="") -> (s? t:f=w377:string)
        n118 = call <vilib>:"Add State(s) to Queue__JKI_lib_State_Machine.vi"("State(s) in (\"\")"=w377, "State(s) at Back (\"\")"="Data: Cleanup\nEvents: Unregister\nExit") -> ("States Out"=w375:string)  [unwired: 13 in]
        n119 = call <vilib>:"Add State(s) to Queue__JKI_lib_State_Machine.vi"("State(s) in Front (\"\")"=w375, "State(s) in (\"\")"=w384) -> ("States Out"=w383:string)  [unwired: 13 in]
      }
      frame "---------- API ----------" {
        # "Do not put any code in this frame.\n(It is a separator no-op. This category is recommended to use for external API)"
      }
      frame "API: API1" {
        # "If you need to tell who triggered this state , use this string. If it's this case itself, this string is \"\"."
        # "Deal with the parameter if any"
        # "Connect this to return the response of your API"
        # "Copy/Rename this case for your own API"
      }
      frame "---------- DoSth ----------" {
        # "Template Separator\n(You can make a copy of, or modify, this frame)"
        n120 = call <vilib>:"Add State(s) to Queue__JKI_lib_State_Machine.vi"("State(s) in (\"\")"=w398) -> ("States Out"=w397:string)  [unwired: 14 in]
      }
      frame "DoSth: DoA" {
        # "Your code here.\n(You can make a copy of, or modify, this frame)"
        n121 = call <vilib>:"Add State(s) to Queue__JKI_lib_State_Machine.vi"("State(s) in (\"\")"=w404) -> ("States Out"=w403:string)  [unwired: 14 in]
      }
      frame "DoSth: DoB" {
        # "Your code here.\n(You can make a copy of, or modify, this frame)"
        n122 = call <vilib>:"Add State(s) to Queue__JKI_lib_State_Machine.vi"("State(s) in (\"\")"=w410) -> ("States Out"=w409:string)  [unwired: 14 in]
      }
    }
  }
  n123 = call "DataSimulateModule.vi"("Name(\"\" to use uuid)"="DataGen" ("Name(\"\" to use uuid)")) -> ()  [unwired: 11 in]
